vi "Request Notifications.vi"(4 "Ignore Past Updates? (F)":bool, 5 "Return Priority (Normal)":T1=enum."Normal", 6 "Value Changes Only? (T)":bool=TRUE, 7 "Notification Msg (Type)":refnum<class "Notification Msg.lvclass">, 8 "error in (no error)":errorcluster, 9 "Data Type":variant, 10 "Topic Name":string, 11 "IObserver in":refnum<class "IObserver.lvclass">) -> (0 "error out":errorcluster, 3 "IObserver out":refnum<class "IObserver.lvclass">)   [LabVIEW 2015, in "IObserver.lvlib" / "IObserver.lvclass"]
doc: "<License>\nCopyright © 2017 Composed Systems, LLC | All rights reserved\nwww.composed.io\n\nAuthor: Ethan Stern <ethan.stern@composed.io>\n\nThis software is provided \"AS IS\" WITHOUT WARRANTIES, either express or implied, AND IS FOR EDUCATIONAL PURPOSES ONLY.\n</License>"
uses:
  IObserver.lvclass
  Mediator/Transport Messages/Notification Msg/Notification Msg.lvclass
  <vilib>/ActorFramework/Message Enqueuer/Message Priority.ctl
  <vilib>/ActorFramework/Actor/Actor.lvclass/Actor.ctl
  <vilib>/ActorFramework/Message Enqueuer/Message Enqueuer.lvclass/Message Enqueuer.ctl
  IMediator/SubscriptionPolicy/SubscriptionPolicy.lvclass/SubscriptionPolicy.ctl
  IObserver Messages/Subscribe Msg/Subscribe Msg.lvclass/Subscribe Msg.ctl
  <vilib>/ActorFramework/Message Enqueuer/Init from Existing Queue.vi
  <vilib>/ActorFramework/Message Enqueuer/Enqueue.vi
  <vilib>/ActorFramework/Message Priority Queue/Priority Enqueue.vi
  <vilib>/ActorFramework/Message Enqueuer/Message Enqueuer.lvclass
  IMediator/SubscriptionPolicy/SubscriptionPolicy.lvclass
  IObserver Messages/Subscribe Msg/Subscribe Msg.lvclass
  IMediator/SubscriptionRequest/SubscriptionRequest.lvclass
  <vilib>/ActorFramework/Actor/Actor.lvclass
  Mediator/Transport/ActorMessage/ActorMessage.lvclass
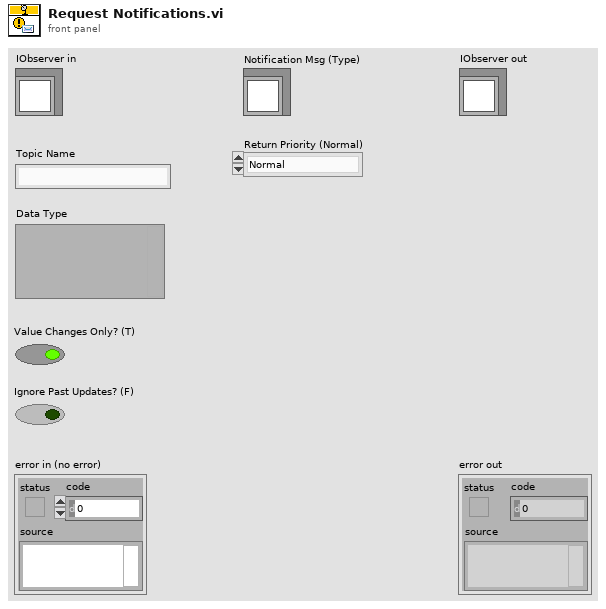
[diagram p1: front panel]
types:
  T1 = typedef "Actor Framework.lvlib/Message Enqueuer.lvclass/Message Priority.ctl" = enum16{"Low", "Normal", "High"}
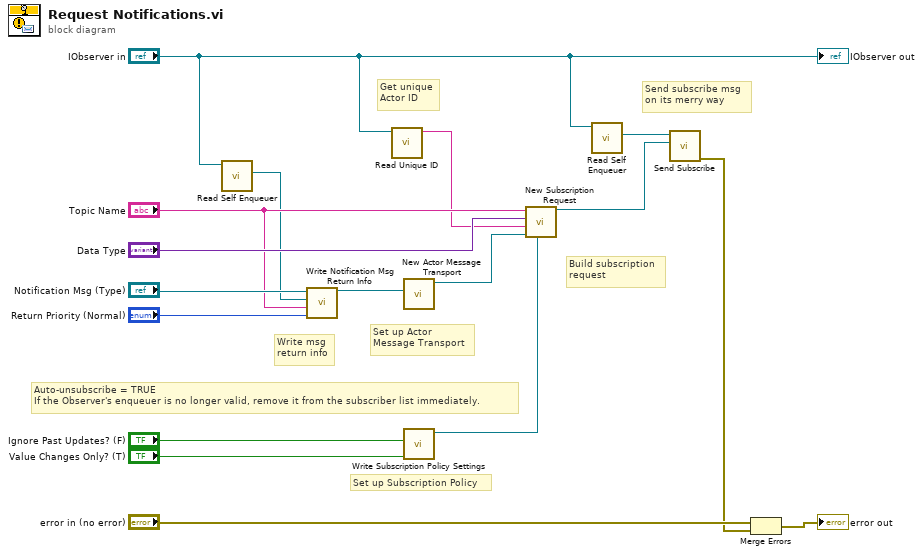
[diagram p0: block diagram]
diagram:
  # "Auto-unsubscribe = TRUE\nIf the Observer's enqueuer is no longer valid, remove it from the subscriber list immediately."
  # "Set up Subscription Policy"
  # "Write msg\nreturn info"
  # "Send subscribe msg\non its merry way"
  # "Build subscription\nrequest"
  # "Get unique\nActor ID"
  # "Set up Actor\nMessage Transport"
  n1 = call <vilib>:"Read Self Enqueuer.vi"("Actor"="IObserver in") -> ("Self Enqueuer"=w5:refnum<class "Message Enqueuer.lvclass">)  [unwired: 10 in]
  n2 = call "Write Notification Msg Return Info.vi"("Return Priority (Normal)"="Return Priority (Normal)", "Topic Name"="Topic Name", "Message Enqueuer in"=w5, "Notification Msg"="Notification Msg (Type)") -> ("Notification Msg Out"=w11:refnum<class "Notification Msg.lvclass">)  [unwired: 7 in]
  n3 = call "Read Unique ID.vi"("IObserver In"="IObserver in") -> ("Unique ID"=w4:string)  [unwired: 10 in]
  n4 = call "New Actor Message Transport.vi"("Desired Notification Msg"=w11) -> ("ActorMessage out"=w16:refnum<class "ActorMessage.lvclass">)  [unwired: 9 in, 1 out]
  n5 = call "Write Subscription Policy Settings.vi"("Value Changes Only? (F)"="Value Changes Only? (T)", "Ignore Past Updates? (F)"="Ignore Past Updates? (F)") -> ("SubscriptionPolicy out"=w3:refnum<class "SubscriptionPolicy.lvclass">)  [unwired: 9 in]
  n6 = call "New Subscription Request.vi"("SubscriptionPolicy"=w3, "Transport"=w16, "Unique Subscriber ID"=w4, "Type"="Data Type", "Topic Name"="Topic Name") -> ("SubscriptionRequest out"=w14:refnum<class "SubscriptionRequest.lvclass">)  [unwired: 6 in]
  n7 = call <vilib>:"Read Self Enqueuer.vi"("Actor"="IObserver in") -> ("Self Enqueuer"=w15:refnum<class "Message Enqueuer.lvclass">)  [unwired: 10 in]
  n8 = call "Send Subscribe.vi"("SubscriptionRequest"=w14, "Message Enqueuer"=w15) -> ("error out"=w12:errorcluster)  [unwired: 8 in, 1 out]
  n9 = Merge Errors("error in (no error)", w12) -> (→"error out":errorcluster)
  "IObserver out" <- "IObserver in"
